vi "FPGA Modular.vi"() -> ()   [LabVIEW 2014]
uses:
  FPGA/SLSC FPGA Inputs.ctl
  <userlib>/_NI SPI IP/FPGA/Controllers/Public/Transfer Settings.ctl
  FPGA/SLSC version.ctl
  FPGA/SLSC FIFO name.ctl
  FPGA/SLSC # of racks.ctl
  FPGA/SLSC SPI Digital IO Lines.ctl
  <vilib>/rvi/Emulation/niFpgaGetClockAttributes.vi
  <vilib>/rvi/Emulation/niFpgaSctlEmulationGetInTimedLoop.vi
  <vilib>/rvi/Emulation/niFpgaEmulationReportErrorSimple.vi
  <vilib>/rvi/interface/RandomDataEmulation/niFpgaRandomDataHandleErrors.vi
  <vilib>/rvi/Emulation/niFpgaCriticalErrorInLSC.vi
  <vilib>/rvi/DataTransferAndStorage/Container/XNode/niFpgaContainer.xnode
  <vilib>/rvi/interface/RandomDataEmulation/nirviRandomDataFpgaReadWriteTemplate.vi
  FPGA/SLSC FPGA Toolkit.lvlib
  <userlib>/_NI SPI IP/FPGA/Controllers/NI SPI IP FPGA.lvlib
panel:
  in  "slsc.# of Racks.4":T1
  in  "slsc.FIFO Name.SPI CMD FIFO":T2
  in  "slsc.version":T3
  in  "settings.SLSC":T4={"SPI PHY Settings"={"Divide Value"=20, "Transfer Length (bits)"=32, "CS Asserted Polarity"=FALSE, "Clock Polarity (CPOL)"=FALSE, "Clock Phase (CPHA)"=FALSE, "Lengthen MISO Setup"=FALSE, "Direction Change Bit"=0, "MOSI Starts as Output"=FALSE, "Tristatable MOSI"=FALSE}, "Sample Rate (S/s)"=10000} {"SPI PHY Settings"."Direction Change Bit" max=64 step=1; "SPI PHY Settings"."Transfer Length (bits)" min=1 max=64 step=1}
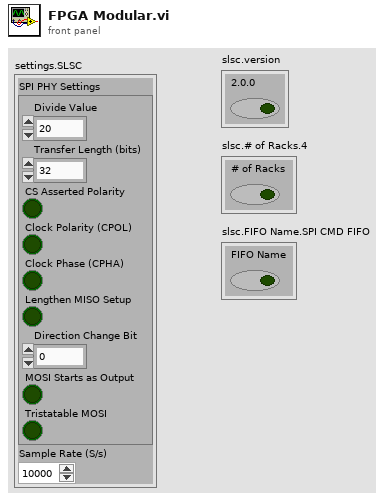
[diagram p1: front panel]
types:
  T1 = typedef "SLSC FPGA Toolkit.lvlib/SLSC # of racks.ctl" = cluster{"# of Racks":bool}
  T2 = typedef "SLSC FPGA Toolkit.lvlib/SLSC FIFO name.ctl" = cluster{"FIFO Name":bool}
  T3 = typedef "SLSC FPGA Toolkit.lvlib/SLSC version.ctl" = cluster{"2.0.0":bool}
  T4 = typedef "SLSC FPGA Toolkit.lvlib/SLSC FPGA Inputs.ctl" = cluster{"SPI PHY Settings":T5, "Sample Rate (S/s)":u32}
  T5 = typedef "NI SPI IP FPGA.lvlib/Transfer Settings.ctl" = cluster{"Divide Value":u8, "Transfer Length (bits)":u8, "CS Asserted Polarity":bool, "Clock Polarity (CPOL)":bool, "Clock Phase (CPHA)":bool, "Lengthen MISO Setup":bool, "Direction Change Bit":u8, "MOSI Starts as Output":bool, "Tristatable MOSI":bool}
  T6 = typedef "SLSC FPGA Toolkit.lvlib/SLSC SPI Digital IO Lines.ctl" = cluster{"SCLK":refnum<k21>, "MISO":refnum<k21>, "MOSI":refnum<k21>, "!Enable":refnum<k21>, "CS Bit 1":refnum<k21>, "CS Bit 2":refnum<k21>, "CS Bit 3":refnum<k21>, "CS Bit 4":refnum<k21>}
  T7 = typedef "SLSC configuration Shared.lvlib/CS Bits.ctl" = cluster{"CS Bit 1":refnum<k21>, "CS Bit 2":refnum<k21>, "CS Bit 3":refnum<k21>, "CS Bit 4":refnum<k21>}
  T8 = typedef "Internal Data (SPI API).ctl" = cluster{"DLU To SPI Engine Data FIFO":refnum<k21>, "SPI Engine to DLU Data FIFO":refnum<k21>, "Data to SPI Engine (Cache) Register":refnum<k21>, "SPI PHY Settings to SPI Engine (Cahche) Register":refnum<k21>}
  T9 = typedef "SPI Digital IO Lines.ctl" = cluster{"SCLK":refnum<k21>, "MISO":refnum<k21>, "MOSI":refnum<k21>, "CS 0":refnum<k21>, "CS 1":refnum<k21>, "CS 2":refnum<k21>, "CS 3":refnum<k21>, "CS 4":refnum<k21>, "CS 5":refnum<k21>}
  T10 = typedef "SLSC FPGA Toolkit.lvlib/SLSC SPI Command.ctl" = cluster{"Chip Select":u8, "SPI PHY Settings":T5, "Data to DAC":u64}
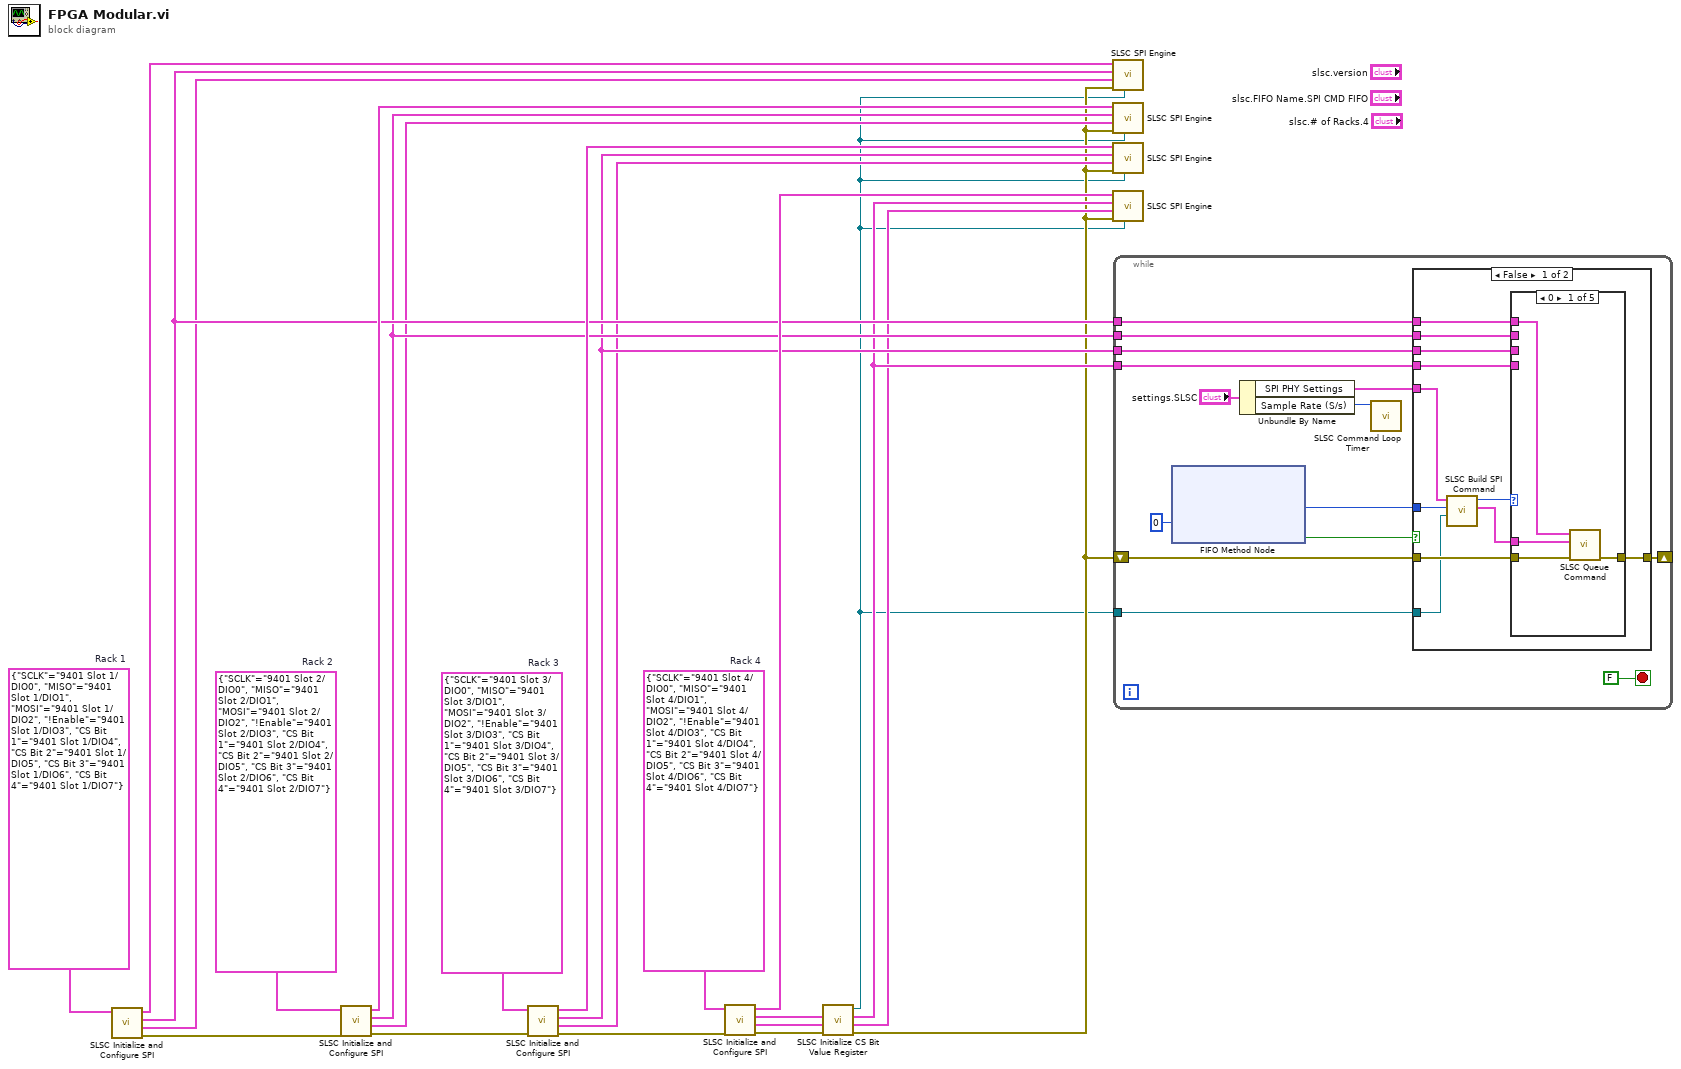
[diagram p0: block diagram]
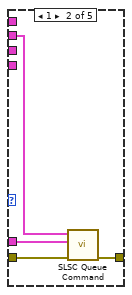
[diagram p2: hidden frame]
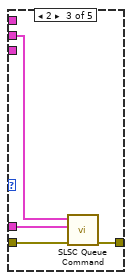
[diagram p3: hidden frame]
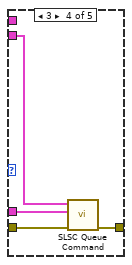
[diagram p4: hidden frame]
diagram:
  w1 = T6 {"SCLK"="9401 Slot 4/DIO0", "MISO"="9401 Slot 4/DIO1", "MOSI"="9401 Slot 4/DIO2", "!Enable"="9401 Slot 4/DIO3", "CS Bit 1"="9401 Slot 4/DIO4", "CS Bit 2"="9401 Slot 4/DIO5", "CS Bit 3"="9401 Slot 4/DIO6", "CS Bit 4"="9401 Slot 4/DIO7"}  # Rack 4
  w2 = T6 {"SCLK"="9401 Slot 3/DIO0", "MISO"="9401 Slot 3/DIO1", "MOSI"="9401 Slot 3/DIO2", "!Enable"="9401 Slot 3/DIO3", "CS Bit 1"="9401 Slot 3/DIO4", "CS Bit 2"="9401 Slot 3/DIO5", "CS Bit 3"="9401 Slot 3/DIO6", "CS Bit 4"="9401 Slot 3/DIO7"}  # Rack 3
  w3 = T6 {"SCLK"="9401 Slot 2/DIO0", "MISO"="9401 Slot 2/DIO1", "MOSI"="9401 Slot 2/DIO2", "!Enable"="9401 Slot 2/DIO3", "CS Bit 1"="9401 Slot 2/DIO4", "CS Bit 2"="9401 Slot 2/DIO5", "CS Bit 3"="9401 Slot 2/DIO6", "CS Bit 4"="9401 Slot 2/DIO7"}  # Rack 2
  w21 = T6 {"SCLK"="9401 Slot 1/DIO0", "MISO"="9401 Slot 1/DIO1", "MOSI"="9401 Slot 1/DIO2", "!Enable"="9401 Slot 1/DIO3", "CS Bit 1"="9401 Slot 1/DIO4", "CS Bit 2"="9401 Slot 1/DIO5", "CS Bit 3"="9401 Slot 1/DIO6", "CS Bit 4"="9401 Slot 1/DIO7"}  # Rack 1
  n1 = call "SLSC Initialize and Configure SPI.vi"("SLSC Chip Select DIO Lines"=w21) -> ("error out"=w20:errorcluster, "CS Bits"=w10:T7, "SPI API References"=w14:T8, "SPI DIO Lines"=w22:T9)  [unwired: 7 in]
  n2 = call "SLSC Initialize and Configure SPI.vi"("error in"=w20, "SLSC Chip Select DIO Lines"=w3) -> ("error out"=w19:errorcluster, "CS Bits"=w9:T7, "SPI API References"=w13:T8, "SPI DIO Lines"=w17:T9)  [unwired: 6 in]
  n3 = call "SLSC Initialize and Configure SPI.vi"("error in"=w19, "SLSC Chip Select DIO Lines"=w2) -> ("error out"=w18:errorcluster, "CS Bits"=w8:T7, "SPI API References"=w12:T8, "SPI DIO Lines"=w16:T9)  [unwired: 6 in]
  n4 = call "SLSC Initialize and Configure SPI.vi"("error in"=w18, "SLSC Chip Select DIO Lines"=w1) -> ("error out"=w6:errorcluster, "CS Bits"=w7:T7, "SPI API References"=w11:T8, "SPI DIO Lines"=w15:T9)  [unwired: 6 in]
  n5 = call "SLSC Initialize CS Bit Value Register.vi"("error in (no error)"=w6) -> ("error out"=w5:errorcluster, "CS Bit Value Register"=w4:refnum<k21>)  [unwired: 9 in]
  n6 = call "SLSC SPI Engine.vi"("CS Bit Value Register"=w4, "error in (no error)"=w5, "CS Bits"=w10, "SPI API References"=w14, "Chip Select DIO Lines"=w22) -> ()  [unwired: 7 in]
  n7 = call "SLSC SPI Engine.vi"("CS Bit Value Register"=w4, "error in (no error)"=w5, "CS Bits"=w9, "SPI API References"=w13, "Chip Select DIO Lines"=w17) -> ()  [unwired: 7 in]
  n8 = call "SLSC SPI Engine.vi"("CS Bit Value Register"=w4, "error in (no error)"=w5, "CS Bits"=w8, "SPI API References"=w12, "Chip Select DIO Lines"=w16) -> ()  [unwired: 7 in]
  n9 = call "SLSC SPI Engine.vi"("CS Bit Value Register"=w4, "error in (no error)"=w5, "CS Bits"=w7, "SPI API References"=w11, "Chip Select DIO Lines"=w15) -> ()  [unwired: 7 in]
  n10 = while {
    tunnel: w14 -> [w34]
    tunnel: w13 -> [w33]
    tunnel: w12 -> [w32]
    tunnel: w11 -> [w31]
    shift-right: [w29] -> _
    shift-left: w5 -> [w30]
    tunnel: w4 -> [w23]
    stop <- FALSE stop-if-true
    n11 = xnode ("FIFO Method Node")("Timeout"=0) -> ("Element"=w35:u64, "Timed Out?"=w27:bool)  [unwired: 1 in, 1 out]
    n12 = Unbundle By Name("settings.SLSC") -> ("SPI PHY Settings"=w25:T5, "Sample Rate (S/s)"=w24:u32)
    n13 = call "SLSC Command Loop Timer.vi"("inputs.Sample Rate (S/s)"=w24) -> ()  [unwired: 8 in, 3 out]
    n14 = case shown="False" w27 {
      tunnel: w35 -> [w47 _]
      tunnel: w25 -> [w46 _]
      tunnel: w34 -> [w43 _]
      tunnel: w33 -> [w42 _]
      tunnel: w32 -> [w41 _]
      tunnel: w31 -> [w40 _]
      tunnel: w30 -> [w39 w65]
      tunnel: [w38 w65] -> w29
      tunnel: w23 -> [w37 _]
      frame False {
        n15 = call "SLSC Build SPI Command.vi"("CS Bit Value Register"=w37, "SPI CMD FIFO Element"=w47, "SPI PHY Settings"=w46) -> ("SLSC SPI Command"=w44:T10, "Rack #"=w45:u8)  [unwired: 7 in]
        n16 = case shown="0" w45 {
          tunnel: w44 -> [w51 w55 w59 w63 _]
          tunnel: w43 -> [w50 _ _ _ _]
          tunnel: w42 -> [_ w52 _ _ _]
          tunnel: w41 -> [_ _ w56 _ _]
          tunnel: w40 -> [_ _ _ w60 _]
          tunnel: w39 -> [w49 w54 w58 w62 w64]
          tunnel: [w48 w53 w57 w61 w64] -> w38
          frame 0 {
            n17 = call "SLSC Queue Command.vi"("error in"=w49, "SLSC SPI Command"=w51, "SPI API References"=w50) -> ("error out"=w48:errorcluster)  [unwired: 6 in, 2 out]
          }
          frame 1 {
            n18 = call "SLSC Queue Command.vi"("error in"=w54, "SLSC SPI Command"=w55, "SPI API References"=w52) -> ("error out"=w53:errorcluster)  [unwired: 6 in, 2 out]
          }
          frame 2 {
            n19 = call "SLSC Queue Command.vi"("error in"=w58, "SLSC SPI Command"=w59, "SPI API References"=w56) -> ("error out"=w57:errorcluster)  [unwired: 6 in, 2 out]
          }
          frame 3 {
            n20 = call "SLSC Queue Command.vi"("error in"=w62, "SLSC SPI Command"=w63, "SPI API References"=w60) -> ("error out"=w61:errorcluster)  [unwired: 6 in, 2 out]
          }
          frame Default {
          }
        }
      }
      frame True {
      }
    }
  }
